vi "VISA Write.vi"(8 "error in":errorcluster, 10 "write buffer":string, 11 "VISA resource name":refnum<visa-resource-name>) -> (0 "error out":errorcluster, 2 "return count":u32, 3 "VISA resource name out":refnum<visa-resource-name>)   [LabVIEW 2017, in "DmmPwr Simulator.lvlib"]
uses:
  DmmPwr Simulator.lvlib
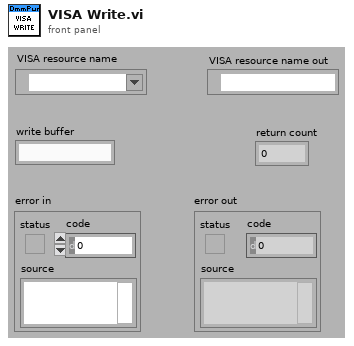
[diagram p1: front panel]
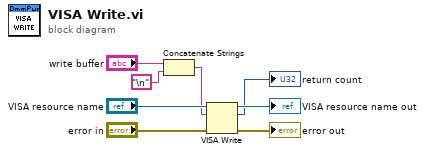
[diagram p0: block diagram]
diagram:
  n1 = Concatenate Strings("write buffer", "\n") -> (w2:string)
  n2 = VISA Write(VISA resource name="VISA resource name", write buffer=w2, error in (no error)="error in") -> (VISA resource name out=→"VISA resource name out":refnum<visa-resource-name>, return count=→"return count":u32, error out=→"error out":errorcluster)
